vi "Sub_SaveTXT.vi"(0 "y_var":dbl[][](array[numeric]), 1 "x_var":dbl[][](array[numeric]), 2 "Validity":i32[](array[numeric]), 3 "DirPath":path) -> ()   [LabVIEW 2014]
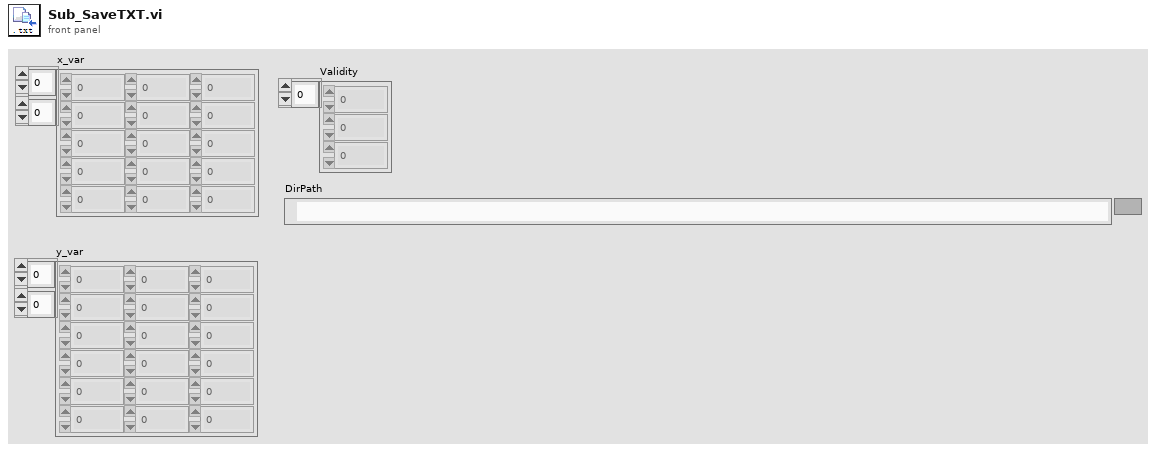
[diagram p1: front panel]
types:
  T1 = enum16{"open", "replace", "create", "open or create", "replace or create", "replace or create with confirmation"}
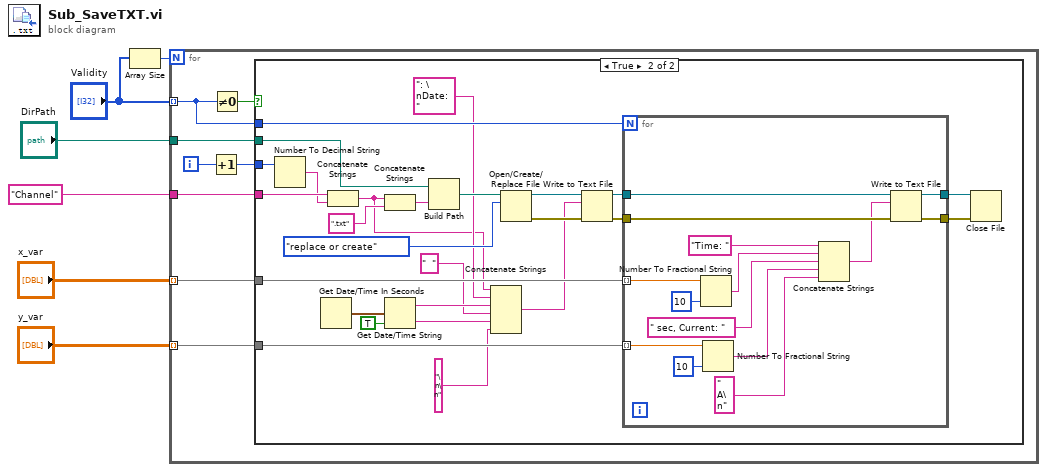
[diagram p0: block diagram]
diagram:
  n1 = Array Size(array="Validity") -> (size(s)=w6:i32)
  n2 = for {
    N: w6 -> [_]
    tunnel: "Validity" -> [w7] mode=indexing
    tunnel: "DirPath" -> [w13]
    tunnel: "Channel" -> [w10]
    tunnel: "x_var" -> [w9] mode=indexing
    tunnel: "y_var" -> [w8] mode=indexing
    i -> [w12]
    n3 = Increment(x=w12) -> (x+1=w11:i32)
    n4 = Not Equal To 0?(x=w7) -> (x != 0?=w14:bool)
    n5 = case shown="True" w14 {
      tunnel: w13 -> [_ w35]
      tunnel: w11 -> [_ w39]
      tunnel: w10 -> [_ w38]
      tunnel: w9 -> [_ w33]
      tunnel: w8 -> [_ w32]
      tunnel: w7 -> [_ w34]
      frame False {
      }
      frame True {
        n6 = Number To Decimal String(number=w39) -> (decimal integer string=w37:string)  [unwired: 1 in]
        n7 = Get Date/Time In Seconds() -> (seconds since 1Jan1904=w24:timestamp)
        n8 = Concatenate Strings(w38, w37) -> (w15:string)
        n9 = Concatenate Strings(w15, ".txt" ("string")) -> (w17:string)
        n10 = Get Date/Time String(seconds (now)=w24, want seconds? (F)=TRUE) -> (date string=w22:string, time string=w20:string)  [unwired: 1 in]
        n11 = Build Path(base path=w35, name or relative path=w17) -> (appended path=w36:path)
        n12 = Concatenate Strings(w15, ": \nDate: " ("string"), w22, "  " ("string"), w20, "\n\n" ("string")) -> (w25:string)
        n13 = Open/Create/Replace File(file path (use dialog)=w36, operation (0:open)=T1."replace or create") -> (refnum out=w27:refnum<file>, error out=w26:errorcluster)  [unwired: 4 in, 1 out]
        n14 = Write to Text File(file (use dialog)=w27, text=w25, error in=w26) -> (refnum out=w29:refnum<file>, error out=w28:errorcluster)  [unwired: 1 in, 1 out]
        n15 = for {
          N: w34 -> [_]
          tunnel: w29 -> [w50]
          tunnel: w28 -> [w49]
          tunnel: w33 -> [w54] mode=indexing
          tunnel: w32 -> [w51] mode=indexing
          tunnel: [w48] -> w31
          tunnel: [w47] -> w30
          n16 = Number To Fractional String(number=w54, precision (6)=i16 10) -> (F-format string=w45:string)  [unwired: 2 in]
          n17 = Number To Fractional String(number=w51, precision (6)=i16 10) -> (F-format string=w43:string)  [unwired: 2 in]
          n18 = Concatenate Strings("Time: ", w45, " sec, Current: ", w43, " A\n") -> (w41:string)
          n19 = Write to Text File(file (use dialog)=w50, text=w41, error in=w49) -> (refnum out=w48:refnum<file>, error out=w47:errorcluster)  [unwired: 1 in, 1 out]
        }
        n20 = Close File(refnum=w31, error in=w30) -> ()  [unwired: 2 out]
      }
    }
  }
